vi "userauth_keyboard_interactive.vi"() -> ()   [LabVIEW 2013]
doc: "Illustrates how to authenticate using keyboard-interactive authentication."
uses:
  libssh2/libssh2_init_default.vi
  libssh2/libssh2_session_handshake_tcp.vi
  libssh2/libssh2.lvlib
panel:
  out "authenticated":bool
  in  "username":string
  in  "hostname":string="localhost"
  out "error out":errorcluster
  # "This will be TRUE if authentication is successful."
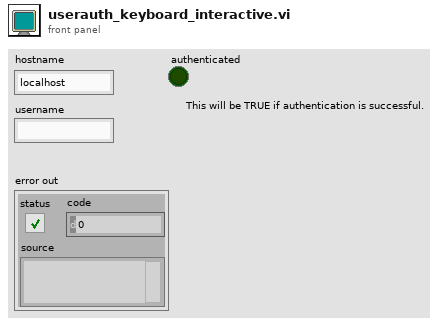
[diagram p1: front panel]
types:
  T1 = typedef "libssh2.lvlib/Session Refnum.ctl" = refnum<k1>
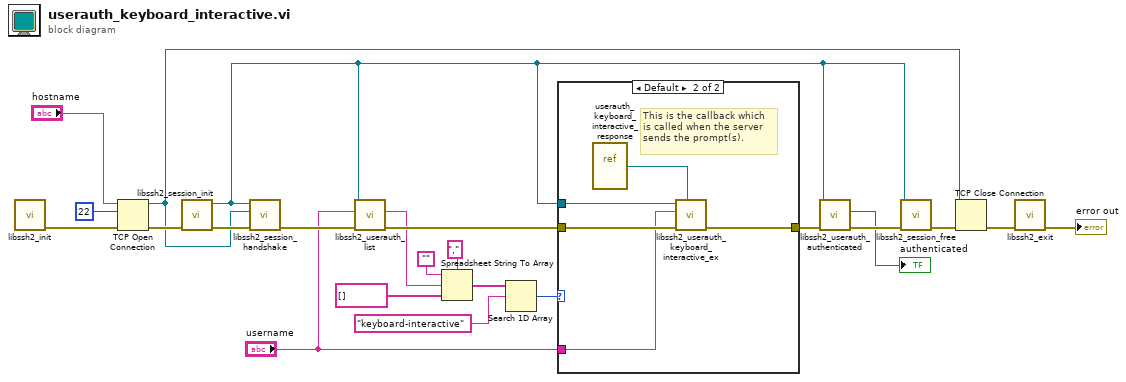
[diagram p0: block diagram]
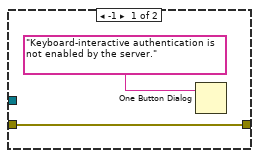
[diagram p2: hidden frame]
diagram:
  n1 = call-poly "libssh2_init.vi"() -> ("error out"=w23:errorcluster)  [unwired: 11 in]
  n2 = TCP Open Connection(address="hostname", remote port or service name=u16 22, error in (no error)=w23) -> (connection ID=w15:refnum<k5>, error out=w16:errorcluster)  [unwired: 2 in]
  n3 = call "libssh2_session_init.vi"("error in (no error)"=w16) -> ("error out"=w18:errorcluster, "session"=w2:T1)  [unwired: 9 in]
  n4 = call-poly "libssh2_session_handshake.vi"("error in (no error)"=w18, "tcp connection"=w15, "session"=w2) -> ("error out"=w14:errorcluster)  [unwired: 8 in]
  n5 = call "libssh2_userauth_list.vi"("error in (no error)"=w14, "username"="username", "session"=w2) -> ("error out"=w10:errorcluster, "supported authentication schemes"=w3:string)  [unwired: 7 in]
  n6 = Spreadsheet String To Array(delimiter (Tab)=",", format string="", spreadsheet string=w3, array type (2D Dbl)=string[] []) -> (array=w5:string[])
  n7 = Search 1D Array(1D array=w5, element="keyboard-interactive") -> (index of element=w1:i32)  [unwired: 1 in]
  n8 = case shown="Default" w1 {
    tunnel: [w25 w30] -> w13
    tunnel: w10 -> [w25 w28]
    tunnel: "username" -> [_ w27]
    tunnel: w2 -> [_ w26]
    frame -1 {
      n9 = One Button Dialog(message="Keyboard-interactive authentication is not enabled by the server.") -> ()  [unwired: 1 in, 1 out]
    }
    frame Default {
      # "This is the callback which\nis called when the server\nsends the prompt(s)."
      n10 = vi-ref "userauth_keyboard_interactive_response.vi"() -> (w29:refnum<vi>)
      n11 = call "libssh2_userauth_keyboard_interactive_ex.vi"("response"=w29, "error in (no error)"=w28, "username"=w27, "session"=w26) -> ("error out"=w30:errorcluster)  [unwired: 7 in]
    }
  }
  n12 = call "libssh2_userauth_authenticated.vi"("error in (no error)"=w13, "session"=w2) -> ("error out"=w12:errorcluster, "authenticated"=→"authenticated":bool)  [unwired: 8 in]
  n13 = call "libssh2_session_free.vi"("error in (no error)"=w12, "session"=w2) -> ("error out"=w17:errorcluster)  [unwired: 9 in]
  n14 = TCP Close Connection(connection ID=w15, error in (no error)=w17) -> (error out=w20:errorcluster)  [unwired: 1 in, 1 out]
  n15 = call "libssh2_exit.vi"("error in (no error)"=w20) -> ("error out"=→"error out":errorcluster)  [unwired: 10 in]
